vi "GaussianRowLocation.vi"(11 "Comments":string) -> (3 "RowXPosition":dbl)   [LabVIEW 2022 SP3]
panel:
  out "ChannelStrings":string[](array[string])
  out "error out":errorcluster
  in  "error in":errorcluster
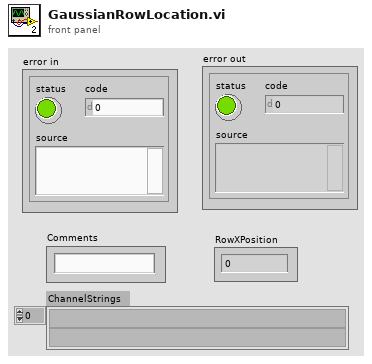
[diagram p1: front panel]
types:
  T1 = enum16{"open", "replace", "create", "open or create", "replace or create", "replace or create with confirmation"}
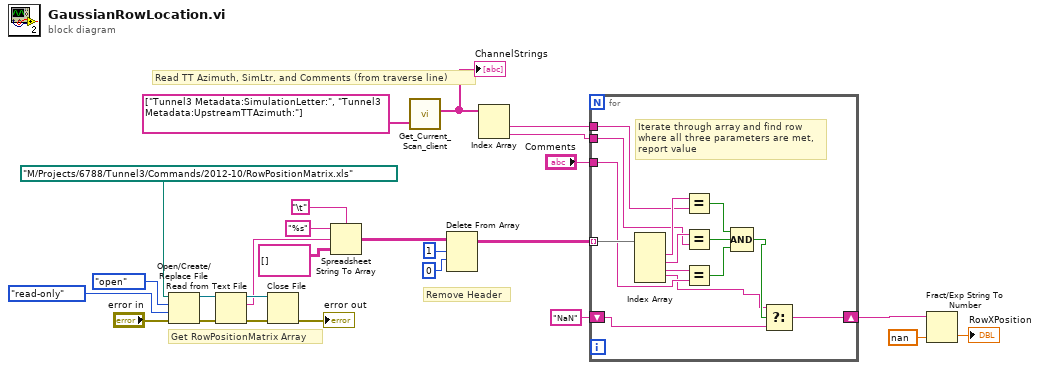
[diagram p0: block diagram]
diagram:
  # "Read TT Azimuth, SimLtr, and Comments (from traverse line)"
  # "Get RowPositionMatrix Array"
  # "Remove Header"
  n1 = Open/Create/Replace File(file path (use dialog)=path "M:/Projects/6788/Tunnel3/Commands/2012-10/RowPositionMatrix.xls", error in="error in", operation (0:open)=T1."open", access (0:read/write)=enum16{"read/write", "read-only", "write-only"}."read-only") -> (refnum out=w20:refnum<file>, error out=w21:errorcluster)  [unwired: 2 in, 1 out]
  n2 = Read from Text File(file (use dialog)=w20, error in=w21) -> (refnum out=w18:refnum<file>, text=w16:string, error out=w19:errorcluster)  [unwired: 2 in, 1 out]
  n3 = Close File(refnum=w18, error in=w19) -> (error out=→"error out":errorcluster)  [unwired: 1 out]
  n4 = Spreadsheet String To Array(delimiter (Tab)="\t", format string="%s", spreadsheet string=w16, array type (2D Dbl)=string[][] []) -> (array=w12:string[][])
  n5 = call "Get_Current_Scan_client.vi"("multipleChannels"=string[] ["Tunnel3 Metadata:SimulationLetter:", "Tunnel3 Metadata:UpstreamTTAzimuth:"] ("ADAM Ch Names")) -> ("String values"=w5:string[])  [unwired: 1 in, 3 out]
  "ChannelStrings" <- w5
  n6 = Delete From Array(array=w12, length=1, index (row)=0) -> (array with subset deleted=w9:string[][])  [unwired: 1 in, 1 out]
  n7 = Index Array(array=w5) -> (element #1=w7:string, element #2=w6:string)  [unwired: 2 in]
  n8 = for {
    tunnel: w9 -> [w40] mode=indexing
    tunnel: "Comments" -> [w34]
    tunnel: w7 -> [w38]
    tunnel: w6 -> [w36]
    shift-right: [w28] -> w2
    shift-left: "NaN" -> [w27]
    # "Iterate through array and find row where all three parameters are met, report value"
    n9 = Index Array(array=w40) -> (element #1=w39:string, element #2=w37:string, element #3=w35:string, element #4=w29:string)  [unwired: 4 in]
    n10 = Equal?(x=w39, y=w38) -> (x = y?=w33:bool)
    n11 = Equal?(x=w37, y=w36) -> (x = y?=w32:bool)
    n12 = Equal?(x=w35, y=w34) -> (x = y?=w31:bool)
    n13 = Compound Arithmetic op=AND(w33, w32, w31) -> (w30:bool)
    n14 = Select(t=w29, s=w30, f=w27) -> (s? t:f=w28:string)
  }
  n15 = Fract/Exp String To Number(string=w2, default (0 dbl)=nan ("default (0 DBL)")) -> (number=→"RowXPosition":dbl)  [unwired: 2 in, 1 out]
